vi "ClientNTTestInit.vi"(11 "Instance":u32) -> (3 "TestConfig":T1)   [LabVIEW 2019]
uses:
  ClientNTTestConfig.ctl
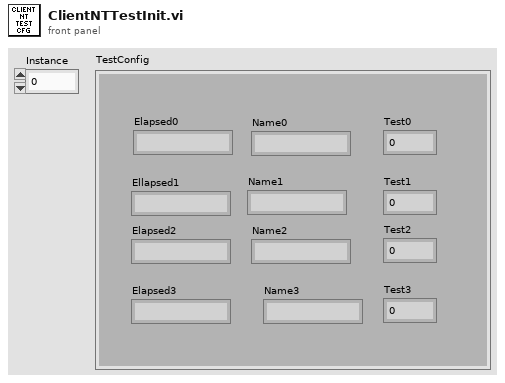
[diagram p1: front panel]
types:
  T1 = typedef "ClientNTTestConfig.ctl" = cluster{"Elapsed0":string, "Name0":string, "Test0":u32, "Ellapsed1":string, "Name1":string, "Test1":u32, "Elapsed2":string, "Name2":string, "Test2":u32, "Elapsed3":string, "Name3":string, "Test3":u32}
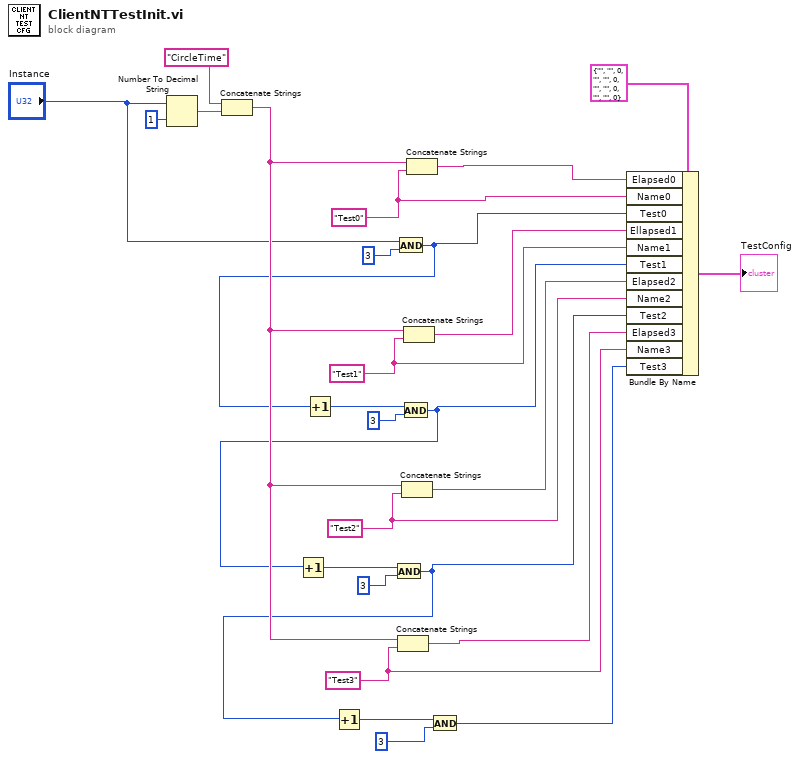
[diagram p0: block diagram]
diagram:
  w2 = "Test3" ("Name")
  w4 = "Test2" ("Name")
  w6 = "Test1" ("Name")
  w8 = "Test0" ("Name")
  n1 = Number To Decimal String(number="Instance", width (-)=i16 1) -> (decimal integer string=w18:string)
  n2 = Concatenate Strings("CircleTime" ("string"), w18) -> (w26:string)
  n3 = And(x="Instance", y=u32 3) -> (x .and. y?=w7:u32)
  n4 = Increment(x=w7) -> (x+1=w21:u32)
  n5 = Concatenate Strings(w26, w2) -> (w11:string)
  n6 = And(x=w21, y=u32 3) -> (x .and. y?=w5:u32)
  n7 = Increment(x=w5) -> (x+1=w23:u32)
  n8 = And(x=w23, y=u32 3) -> (x .and. y?=w3:u32)
  n9 = Increment(x=w3) -> (x+1=w25:u32)
  n10 = Concatenate Strings(w26, w4) -> (w10:string)
  n11 = Concatenate Strings(w26, w6) -> (w9:string)
  n12 = Concatenate Strings(w26, w8) -> (w12:string)
  n13 = And(x=w25, y=u32 3) -> (x .and. y?=w1:u32)
  n14 = Bundle By Name(cluster=T1 {"Elapsed0"="", "Name0"="", "Test0"=0, "Ellapsed1"="", "Name1"="", "Test1"=0, "Elapsed2"="", "Name2"="", "Test2"=0, "Elapsed3"="", "Name3"="", "Test3"=0} ("TestConfig"), "Elapsed0"=w12, "Name0"=w8, "Test0"=w7, "Ellapsed1"=w9, "Name1"=w6, "Test1"=w5, "Elapsed2"=w10, "Name2"=w4, "Test2"=w3, "Elapsed3"=w11, "Name3"=w2, "Test3"=w1) -> (→"TestConfig":T1)
